vi "Evaluate Calibration.vi"(9 "tesla":dbl[unit], 11 "varian in":refnum<class "Varian Magnet.lvclass">) -> (1 "control voltage":dbl, 3 "varian out":refnum<class "Varian Magnet.lvclass">)   [LabVIEW 2009, in "Varian Magnet.lvclass"]
doc: "evaluates the corresponding voltage for a given magnetic field based on the previously extrapolated function."
uses:
  Varian Magnet.lvclass
  Varian Magnet.lvclass/Varian Magnet.ctl
  <vilib>/gmath/NI_Gmath.lvlib
panel:
  out "volts":dbl[](array[numeric]) format="%_6g"
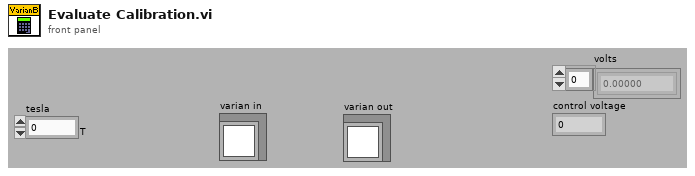
[diagram p1: front panel]
types:
  T1 = typedef "NI_Gmath.lvlib/in_piecewise interp poly control.ctl" = cluster{"x locations":dbl[], "coefficients":dbl[][]}
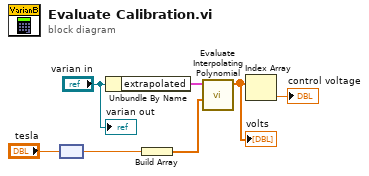
[diagram p0: block diagram]
diagram:
  n1 = node("tesla") -> (w4:dbl)
  n2 = Unbundle By Name("varian in") -> ("extrapolated"=w7:T1)
  n3 = Build Array(w4) -> (w5:dbl[])
  n4 = call <vilib>:"Evaluate Interpolating Polynomial.vi"("xi"=w5, "piecewise polynomial"=w7) -> ("yi"=w2:dbl[])  [unwired: 8 in, 1 out]
  "volts" <- w2
  n5 = Index Array(array=w2) -> (element=→"control voltage":dbl)  [unwired: 1 in]
  "varian out" <- "varian in"
